vi "Message Loop.vi"(8 "error in (no error)":errorcluster) -> (0 "error out":errorcluster)   [LabVIEW 2019, in "DSP.lvclass"]
doc: "Message loop for handling messages pertaining to the acquisition of data from the hardware."
uses:
  DSP/DSP.lvclass
  <vilib>/Utility/error.llb/Error Cluster From Error Code.vi
  <vilib>/ErrorRing/Error Ring.xnode
panel:
  # "message queue"
  # "data queue"
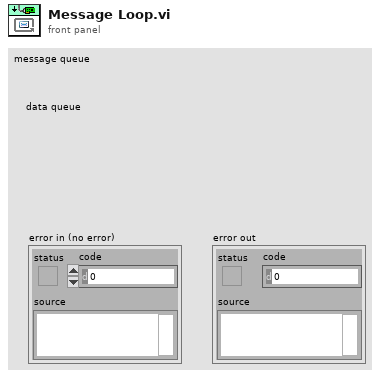
[diagram p1: front panel]
types:
  T1 = typedef "Acquisition.lvlib/Hardware Configuration.ctl" = cluster{"DAQmx Channel":tag, "Max Input":dbl, "Min Input":dbl, "Sample Rate":dbl, "DAQmx Task":refnum<k21>}
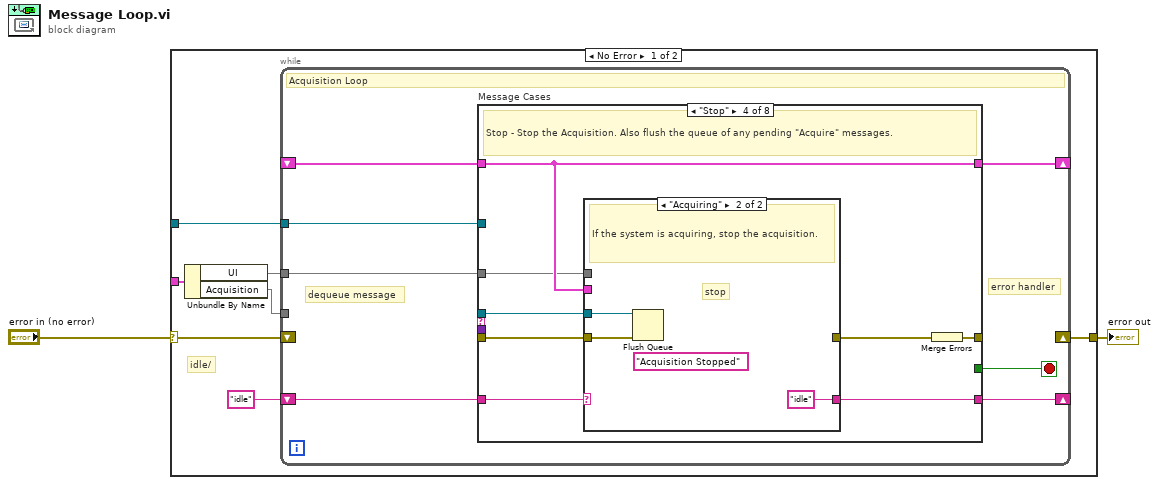
[diagram p0: block diagram]
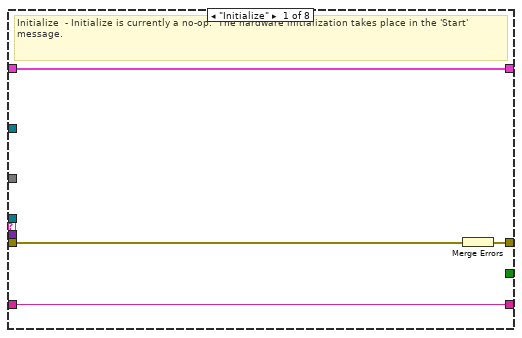
[diagram p2: hidden frame]
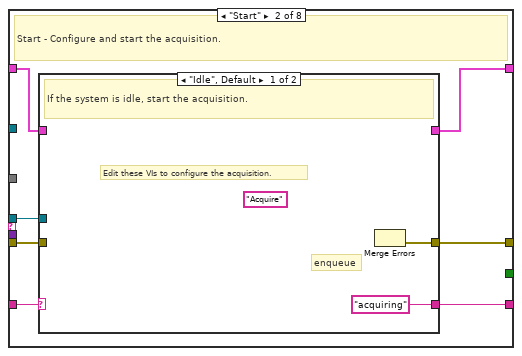
[diagram p3: hidden frame]
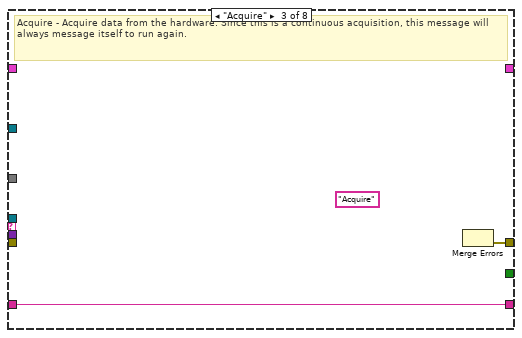
[diagram p5: hidden frame]
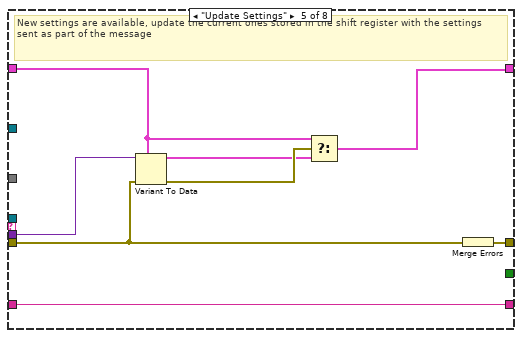
[diagram p7: hidden frame]
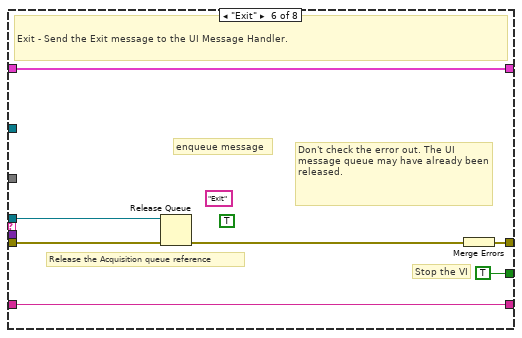
[diagram p8: hidden frame]
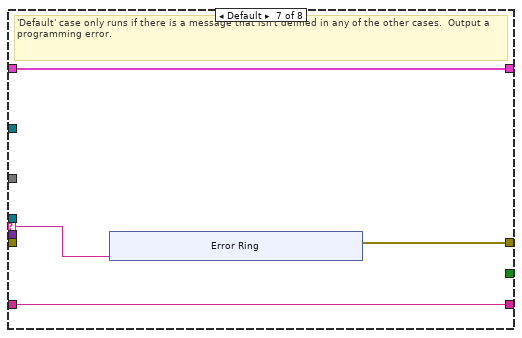
[diagram p9: hidden frame]
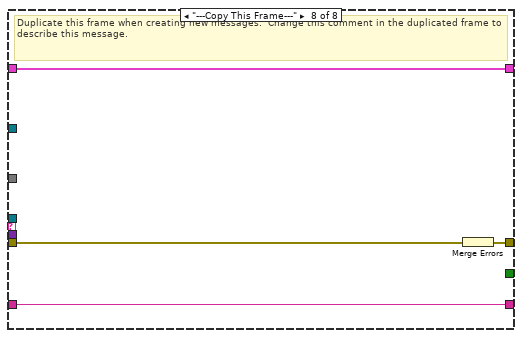
[diagram p10: hidden frame]
diagram:
  n1 = case shown="No Error" "error in (no error)" {
    selector: "error in (no error)" -> [w8 w105]
    tunnel: [w12 _] -> w4
    tunnel: [w10 w105] -> w3
    tunnel: [w6 _] -> w1
    frame No Error {
      # "idle/"
      n2 = Unbundle By Name(w12) -> ("UI"=w7, "Acquisition"=w11)
      n3 = while {
        tunnel: w11 -> [_]
        shift-right: [w23] -> _
        shift-left: [w24] -> w9
        shift-right: [_] -> w10
        shift-left: w8 -> [_]
        tunnel: w7 -> [w15]
        tunnel: w6 -> [w17]
        shift-right: [w13] -> _
        shift-left: "idle" -> [w14]
        stop <- w22 stop-if-true
        # "dequeue message"
        # "error handler"
        # "Acquisition Loop"
        n4 = case "Message Cases" shown="\"Stop\"" w20 {
          selector: [_ _ _ _ _ _ w92 _] -> w20
          tunnel: [_ w32 w54 w60 _ w83 _ _] -> w18
          tunnel: [w27 w33 w53 w62 w74 w86 _ w104] -> w21
          tunnel: [w28 w35 w55 w63 w80 w88 w91 w102] -> w16
          tunnel: w24 -> [w26 w34 w50 w61 w76 w82 w93 w103]
          tunnel: [w26 w31 w51 w61 w75 w82 w93 w103] -> w23
          tunnel: [_ _ _ _ _ TRUE _ _] -> w22
          tunnel: [_ _ _ _ w79 _ _ _] -> w19
          tunnel: w15 -> [_ _ _ w59 _ w87 _ _]
          tunnel: w17 -> [_ _ w48 _ _ _ _ _]
          tunnel: w14 -> [w25 w30 w47 w58 w73 w81 w90 w101]
          tunnel: [w25 w29 w47 w57 w73 w81 w90 w101] -> w13
          frame "Initialize" {
            # "Initialize  - Initialize is currently a no-op.  The hardware initialization takes place in the 'Start' message."
            n5 = Merge Errors(w27) -> (w28:errorcluster)
          }
          frame "Start" {
            # "Start - Configure and start the acquisition."
            n6 = case shown="\"Idle\", Default" w30 {
              selector: w30 -> [_ w44]
              tunnel: [w43 w46] -> w35
              tunnel: w34 -> [w42 w45]
              tunnel: w33 -> [w41 w46]
              tunnel: w32 -> [w40 _]
              tunnel: [w38 w45] -> w31
              tunnel: ["acquiring" w44] -> w29
              frame "Idle", Default {
                w37 = "Acquire" ("Message")
                # "enqueue"
                # "Edit these VIs to configure the acquisition."
                # "If the system is idle, start the acquisition."
                n7 = Merge Errors() -> (w43:errorcluster, w39:errorcluster)  [unwired: 1 in]
              }
              frame "Acquiring" {
                # "The system is already acquiring. Ignore the \"Start\" message."
              }
            }
          }
          frame "Acquire" {
            w49 = "Acquire" ("Message")
            # "Acquire - Acquire data from the hardware. Since this is a continuous acquisition, this message will always message itself to run again."
            n8 = Merge Errors() -> (w55:errorcluster, w52:errorcluster)  [unwired: 1 in]
          }
          frame "Stop" {
            # "Stop - Stop the Acquisition. Also flush the queue of any pending \"Acquire\" messages."
            n9 = case shown="\"Acquiring\"" w58 {
              selector: w58 -> [w65 _]
              tunnel: w62 -> [w64 w72]
              tunnel: w61 -> [_ w71]
              tunnel: w60 -> [_ w69]
              tunnel: w59 -> [_ w68]
              tunnel: [w65 "idle"] -> w57
              tunnel: [w64 _] -> w56
              frame "Idle", Default {
                # "The system is already idle. Ignore the \"Stop\" message."
              }
              frame "Acquiring" {
                w67 = "Acquisition Stopped" ("Message")
                # "stop"
                # "If the system is acquiring, stop the acquisition."
                n10 = Flush Queue(queue=w69, error in (no error)=w72) -> (error out=w70:errorcluster)  [unwired: 2 out]
              }
            }
            n11 = Merge Errors(w56) -> (w63:errorcluster)
          }
          frame "Update Settings" {
            # "New settings are available, update the current ones stored in the shift register with the settings sent as part of the message"
            n12 = Variant To Data(error in=w74, type=w76, Variant=w79) -> (data=w77:T1, error out=w78:errorcluster)
            n13 = Select(t=w76, s=w78, f=w77) -> (s? t:f=w75:T1)
            n14 = Merge Errors(w74) -> (w80:errorcluster)
          }
          frame "Exit" {
            w85 = TRUE
            (unwired) "Exit" ("Message")
            # "enqueue message"
            # "Don't check the error out. The UI message queue may have already been released."
            # "Release the Acquisition queue reference"
            # "Stop the VI"
            # "Exit - Send the Exit message to the UI Message Handler."
            n15 = Release Queue(queue=w83, error in (no error)=w86) -> (error out=w84:errorcluster)  [unwired: 1 in, 2 out]
            n16 = Merge Errors(w84) -> (w88:errorcluster)
          }
          frame Default {
            # "'Default' case only runs if there is a message that isn't defined in any of the other cases.  Output a programming error."
            n17 = xnode "Error Ring"("parameter 0"=w92) -> ("error out"=w91:errorcluster)
          }
          frame "---Copy This Frame---" {
            # "Duplicate this frame when creating new messages.  Change this comment in the duplicated frame to describe this message."
            n18 = Merge Errors(w104) -> (w102:errorcluster)
          }
        }
      }
    }
    frame Error {
    }
  }
  "error out" <- w3
